vi "Handle Last Ack Core.vi"(4 "error in (no error)":errorcluster, 6 "Last Ack":refnum<class "Last Ack.lvclass">, 7 "EmulatorActor in":refnum<class "EmulatorActor.lvclass">) -> (0 "error out":errorcluster, 3 "EmulatorActor out":refnum<class "EmulatorActor.lvclass">)   [LabVIEW 2019, in "EmulatorActor.lvlib" / "EmulatorActor.lvclass"]
doc: "(<B>Filename</B>: Actor Framework.lvlib:Actor.lvclass:Handle Last Ack Core.vi)\n\nDefines how the caller actor responds to the Last Ack message from a nested actor. The Last Ack message is the final message a nested actor sends to its caller before it shuts down. The message contains information about the final state of the nested actor.\n\nBy default, this method does nothing except return any error the nested actor sent. A descendant class may override this method to define behavior."
uses:
  EmulatorActor.lvclass
  <vilib>/ActorFramework/LastAck/Last Ack.lvclass
  C:/Program Files (x86)/National Instruments/LabVIEW 2019/vi.lib/ActorFramework/Actor/Actor.lvclass
  EmulatorActor.lvclass/EmulatorActor.ctl
  DigitiserActor/DigitiserActor/DigitiserActor.lvclass
  <vilib>/ActorFramework/Actor/Actor.lvclass
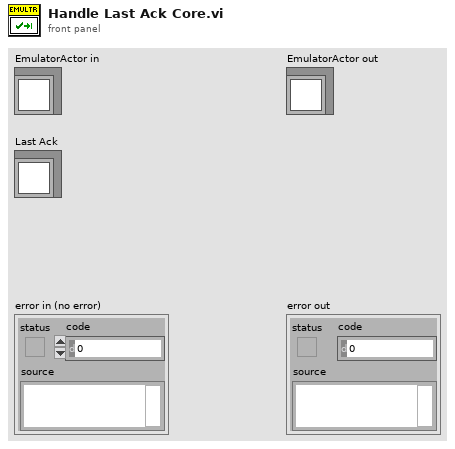
[diagram p1: front panel]
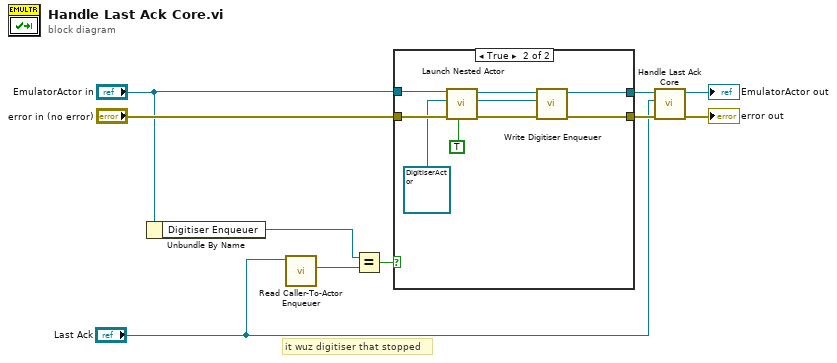
[diagram p0: block diagram]
diagram:
  # "it wuz digitiser that stopped"
  n1 = Unbundle By Name("EmulatorActor in") -> ("Digitiser Enqueuer"=w5:refnum<class "Message Enqueuer.lvclass">)
  n2 = call <vilib>:"Read Caller-To-Actor Enqueuer.vi"("Last Ack"="Last Ack") -> ("Caller-to-Actor Enqueuer"=w6:refnum<class "Message Enqueuer.lvclass">)  [unwired: 10 in]
  n3 = Equal?(x=w5, y=w6) -> (x = y?=w4:bool)
  n4 = case shown="True" w4 {
    tunnel: "error in (no error)" -> [w12 w20]
    tunnel: [w12 w16] -> w7
    tunnel: "EmulatorActor in" -> [w11 w21]
    tunnel: [w11 w14] -> w2
    frame False {
    }
    frame True {
      n5 = call <vilib>:"Launch Nested Actor.vi"("Open Actor Core front panel? (F)"=TRUE, "error in (no error)"=w20, "Nested Actor"=refnum<class "DigitiserActor.lvclass"> refnum ("DigitiserActor.lvlib:DigitiserActor.lvclass"), "Caller Actor in"=w21) -> ("error out"=w19:errorcluster, "Nested Actor's Enqueuer"=w13:refnum<class "Message Enqueuer.lvclass">, "Caller Actor out"=w15:refnum<class "EmulatorActor.lvclass">)  [unwired: 5 in]
      n6 = call "Write Digitiser Enqueuer.vi"("error in (no error)"=w19, "Actor Framework:Message Enqueuer"=w13, "EmulatorActor in"=w15) -> ("error out"=w16:errorcluster, "EmulatorActor out"=w14:refnum<class "EmulatorActor.lvclass">)  [unwired: 7 in]
    }
  }
  n7 = call-parent "Handle Last Ack Core.vi"("error in (no error)"=w7, "Last Ack"="Last Ack", "Actor in"=w2) -> ("error out"=→"error out":errorcluster, "Actor out"=→"EmulatorActor out":refnum<class "EmulatorActor.lvclass">)  [unwired: 3 in]
